vi "StartAsyncEngine.vi"(8 "error in (no error)":errorcluster, 10 "AsyncDVR":refnum<data-value>, 11 "MicronGRPCClient in":refnum<class "MicronGRPCClient.lvclass">) -> (0 "error out":errorcluster, 3 "MicronGRPCClient out":refnum<class "MicronGRPCClient.lvclass">)   [LabVIEW 2019, in "MicronGRPCClient.lvclass"]
uses:
  MicronGRPCClient.lvclass
  Typedefs/AsyncCluster.ctl
  <vilib>/SLL Toolkit/SLL Queued State Machine/Queue Driver/Typedefs/Queue Type.ctl
  <vilib>/SLL Toolkit/SLL Queued State Machine/SLL QSM.lvlib
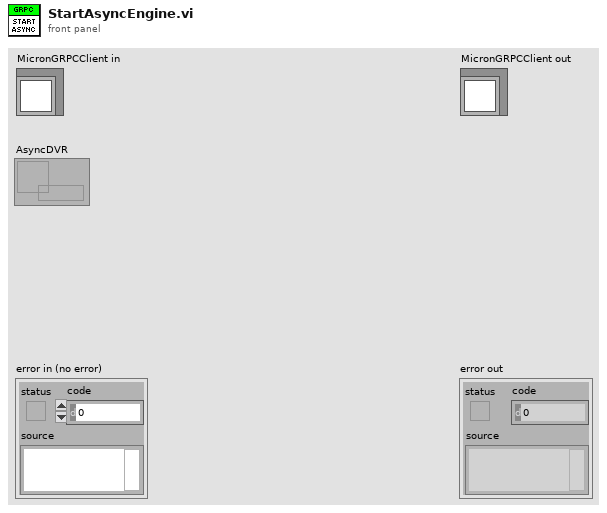
[diagram p1: front panel]
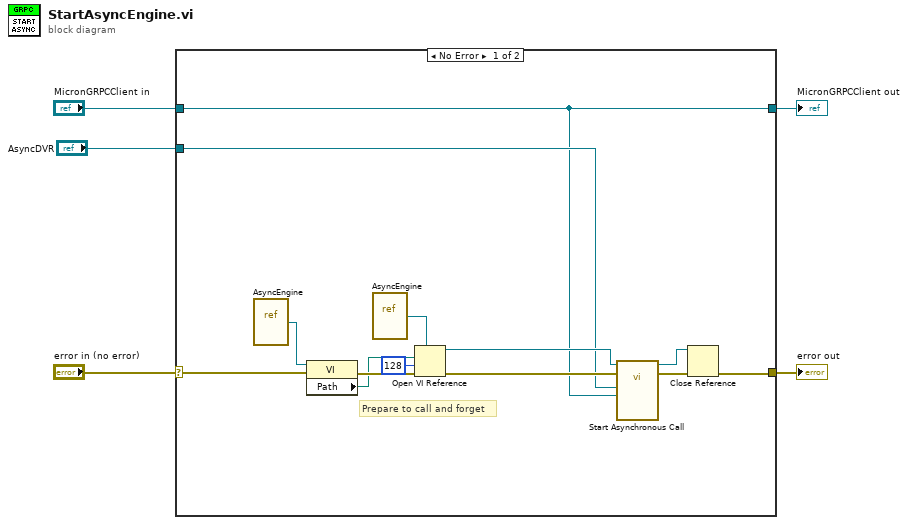
[diagram p0: block diagram]
diagram:
  n1 = case shown="No Error" "error in (no error)" {
    selector: "error in (no error)" -> [w11 w20]
    tunnel: [w8 w20] -> w4
    tunnel: [w6 w19] -> w2
    tunnel: "MicronGRPCClient in" -> [w6 w19]
    tunnel: "AsyncDVR" -> [w7 _]
    frame No Error {
      # "Prepare to call and forget"
      n2 = vi-ref "AsyncEngine.vi"() -> (w14:refnum<vi>)
      n3 = property class="VI"(reference=w14, error in=w11) -> (error out=w16:errorcluster, "Path"=w15:path)  [unwired: 1 out]
      n4 = vi-ref "AsyncEngine.vi"() -> (w12:refnum<vi>)
      n5 = Open VI Reference(type specifier VI Refnum (for type only)=w12, vi path=w15, options=128, error in (no error)=w16) -> (vi reference=w9:refnum<vi>, error out=w10:errorcluster)  [unwired: 2 in]
      n6 = call-by-ref "Start Asynchronous Call"(reference=w9, error in=w10, "MicronGRPCClient in"=w6, "AsyncDVR"=w7) -> (reference out=w17:refnum<vi>, error out=w18:errorcluster)  [unwired: 9 in, 1 out]
      n7 = Close Reference(reference=w17, error in (no error)=w18) -> (error out=w8:errorcluster)
    }
    frame Error {
    }
  }
  "error out" <- w4
  "MicronGRPCClient out" <- w2
